vi "VI Server_Set Text Ring by Item Selected.vi"(7 "Label":string, 8 "error in":errorcluster, 9 "Item":string, 11 "VI Server.RefsCluster":T1 caption="VI Server Cluster") -> (0 "error out":errorcluster, 1 "Control Reference":refnum<vi>, 3 "VI Server Cluster.DUP":T1)   [LabVIEW 2020, in "VI Server Toolkit LV2013.lvlib"]
doc: "Sets value of Text Ring by its item name/selection"
uses:
  VI Server Toolkit LV2013.lvlib
  VI Server_TypeDefs/VI Server_RefsCluster.ctl
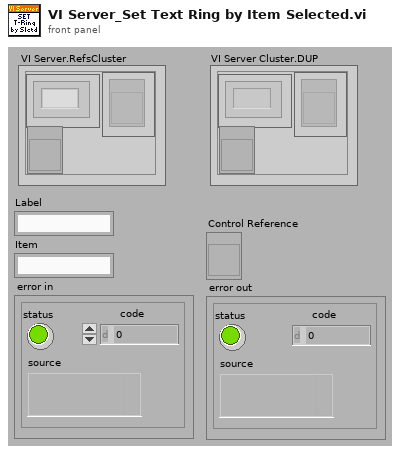
[diagram p1: front panel]
types:
  T1 = typedef "VI Server_RefsCluster.ctl" = cluster{"Labels":string[], "Refs":refnum<vi>[], "VI Ref":refnum<vi>}
  T2 = typedef "LVStringsAndValuesArrayTypeDef_U16.ctl" = cluster{"String":string, "Value":u16}[]
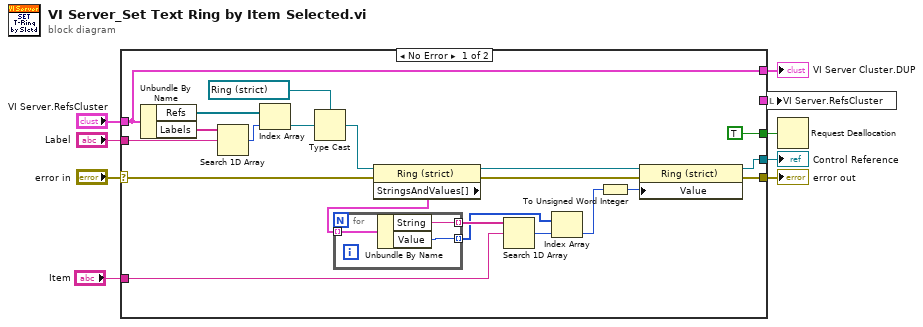
[diagram p0: block diagram]
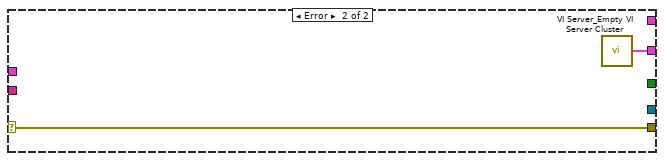
[diagram p2: hidden frame]
diagram:
  n1 = case shown="No Error" "error in" {
    selector: "error in" -> [w24 w35]
    tunnel: "Label" -> [w29 _]
    tunnel: "VI Server.RefsCluster" -> [w11 _]
    tunnel: [w21 w35] -> w9
    tunnel: [w18 _] -> w5
    tunnel: "Item" -> [w23 _]
    tunnel: [w11 _] -> w3
    tunnel: [TRUE _] -> w2
    tunnel: [_ w34] -> w1
    frame No Error {
      n2 = Unbundle By Name(w11) -> ("Refs"=w27:refnum<vi>[], "Labels"=w30:string[])
      n3 = Search 1D Array(1D array=w30, element=w29) -> (index of element=w28:i32)  [unwired: 1 out]
      n4 = Index Array(array=w27, index=w28) -> (element=w26:refnum<vi>)
      n5 = Type Cast(type=refnum<vi> refnum ("Ring"), x=w26) -> (*(type *) &x=w19:refnum<vi>)
      n6 = property class="Ring (strict)"(reference=w19, error in=w24) -> (reference out=w20:refnum<vi>, error out=w22:errorcluster, "StringsAndValues[]"=w16:T2)
      n7 = for {
        tunnel: w16 -> [w33] mode=indexing
        tunnel: [w32] -> w15 mode=indexing
        tunnel: [w31] -> w14 mode=indexing
        n8 = Unbundle By Name(w33) -> ("String"=w32:string, "Value"=w31:u16)
      }
      n9 = Search 1D Array(1D array=w15, element=w23) -> (index of element=w13:i32)  [unwired: 1 out]
      n10 = Index Array(array=w14, index=w13) -> (element=w12:u16)
      n11 = To Unsigned Word Integer(number=w12) -> (unsigned 16bit integer=w17:u16)
      n12 = property class="Ring (strict)"(reference=w20, error in=w22, "Value"=w17) -> (reference out=w18:refnum<vi>, error out=w21:errorcluster)
    }
    frame Error {
      n13 = call "VI Server_Empty VI Server Cluster.vi"() -> ("VI Server Cluster"=w34:T1)  [unwired: 7 in]
    }
  }
  "error out" <- w9
  "VI Server Cluster.DUP" <- w3
  "Control Reference" <- w5
  n14 = local write "VI Server.RefsCluster"(w1) -> ()
  n15 = Request Deallocation(w2) -> ()
